vi "Stepper_control_limits.vi"() -> ()   [LabVIEW 2017]
uses:
  <vilib>/Instr/_visa.llb/VISA Configure Serial Port (Instr).vi
panel:
  out "Correction Collar Position":dbl format="%#_3g"
  in  "Load Limits":bool
  in  "Force Stop":bool
  in  "Save Limits":bool
  out "Feedback String":string
  in  "RUN":bool
  in  "Reset Limit":bool
  out "Serial Command":string
  in  "Speed":enum32{"Fine", "Coarse"}(radio)
  in  "Direction":enum32{"Clockwise", "Anticlockwise"}(radio)
  in  "STOP":bool
  out "Second Limit":dbl
  in  "Second Limit":bool
  out "First Limit":dbl
  in  "First Limit":bool
  out "0.17 Position":dbl
  in  "Home":bool
  out "Encoder Position":dbl
  in  "Arduino UNO COM Port":refnum<visa-resource-name>="COM7"
  # "First to Second limit should be set in clockwise sweep"
  # "Do not use unless necessary"
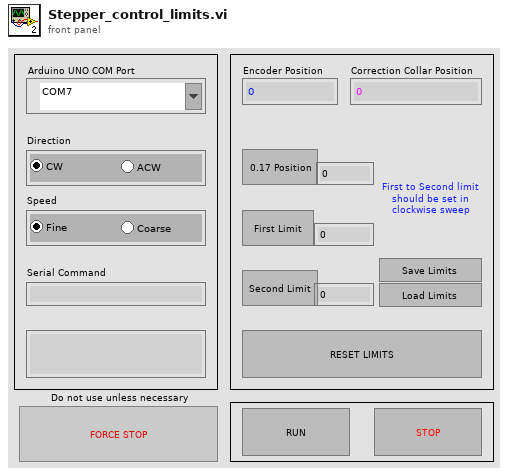
[diagram p1: front panel]
types:
  T1 = enum16{"open", "replace", "create", "open or create", "replace or create", "replace or create with confirmation"}
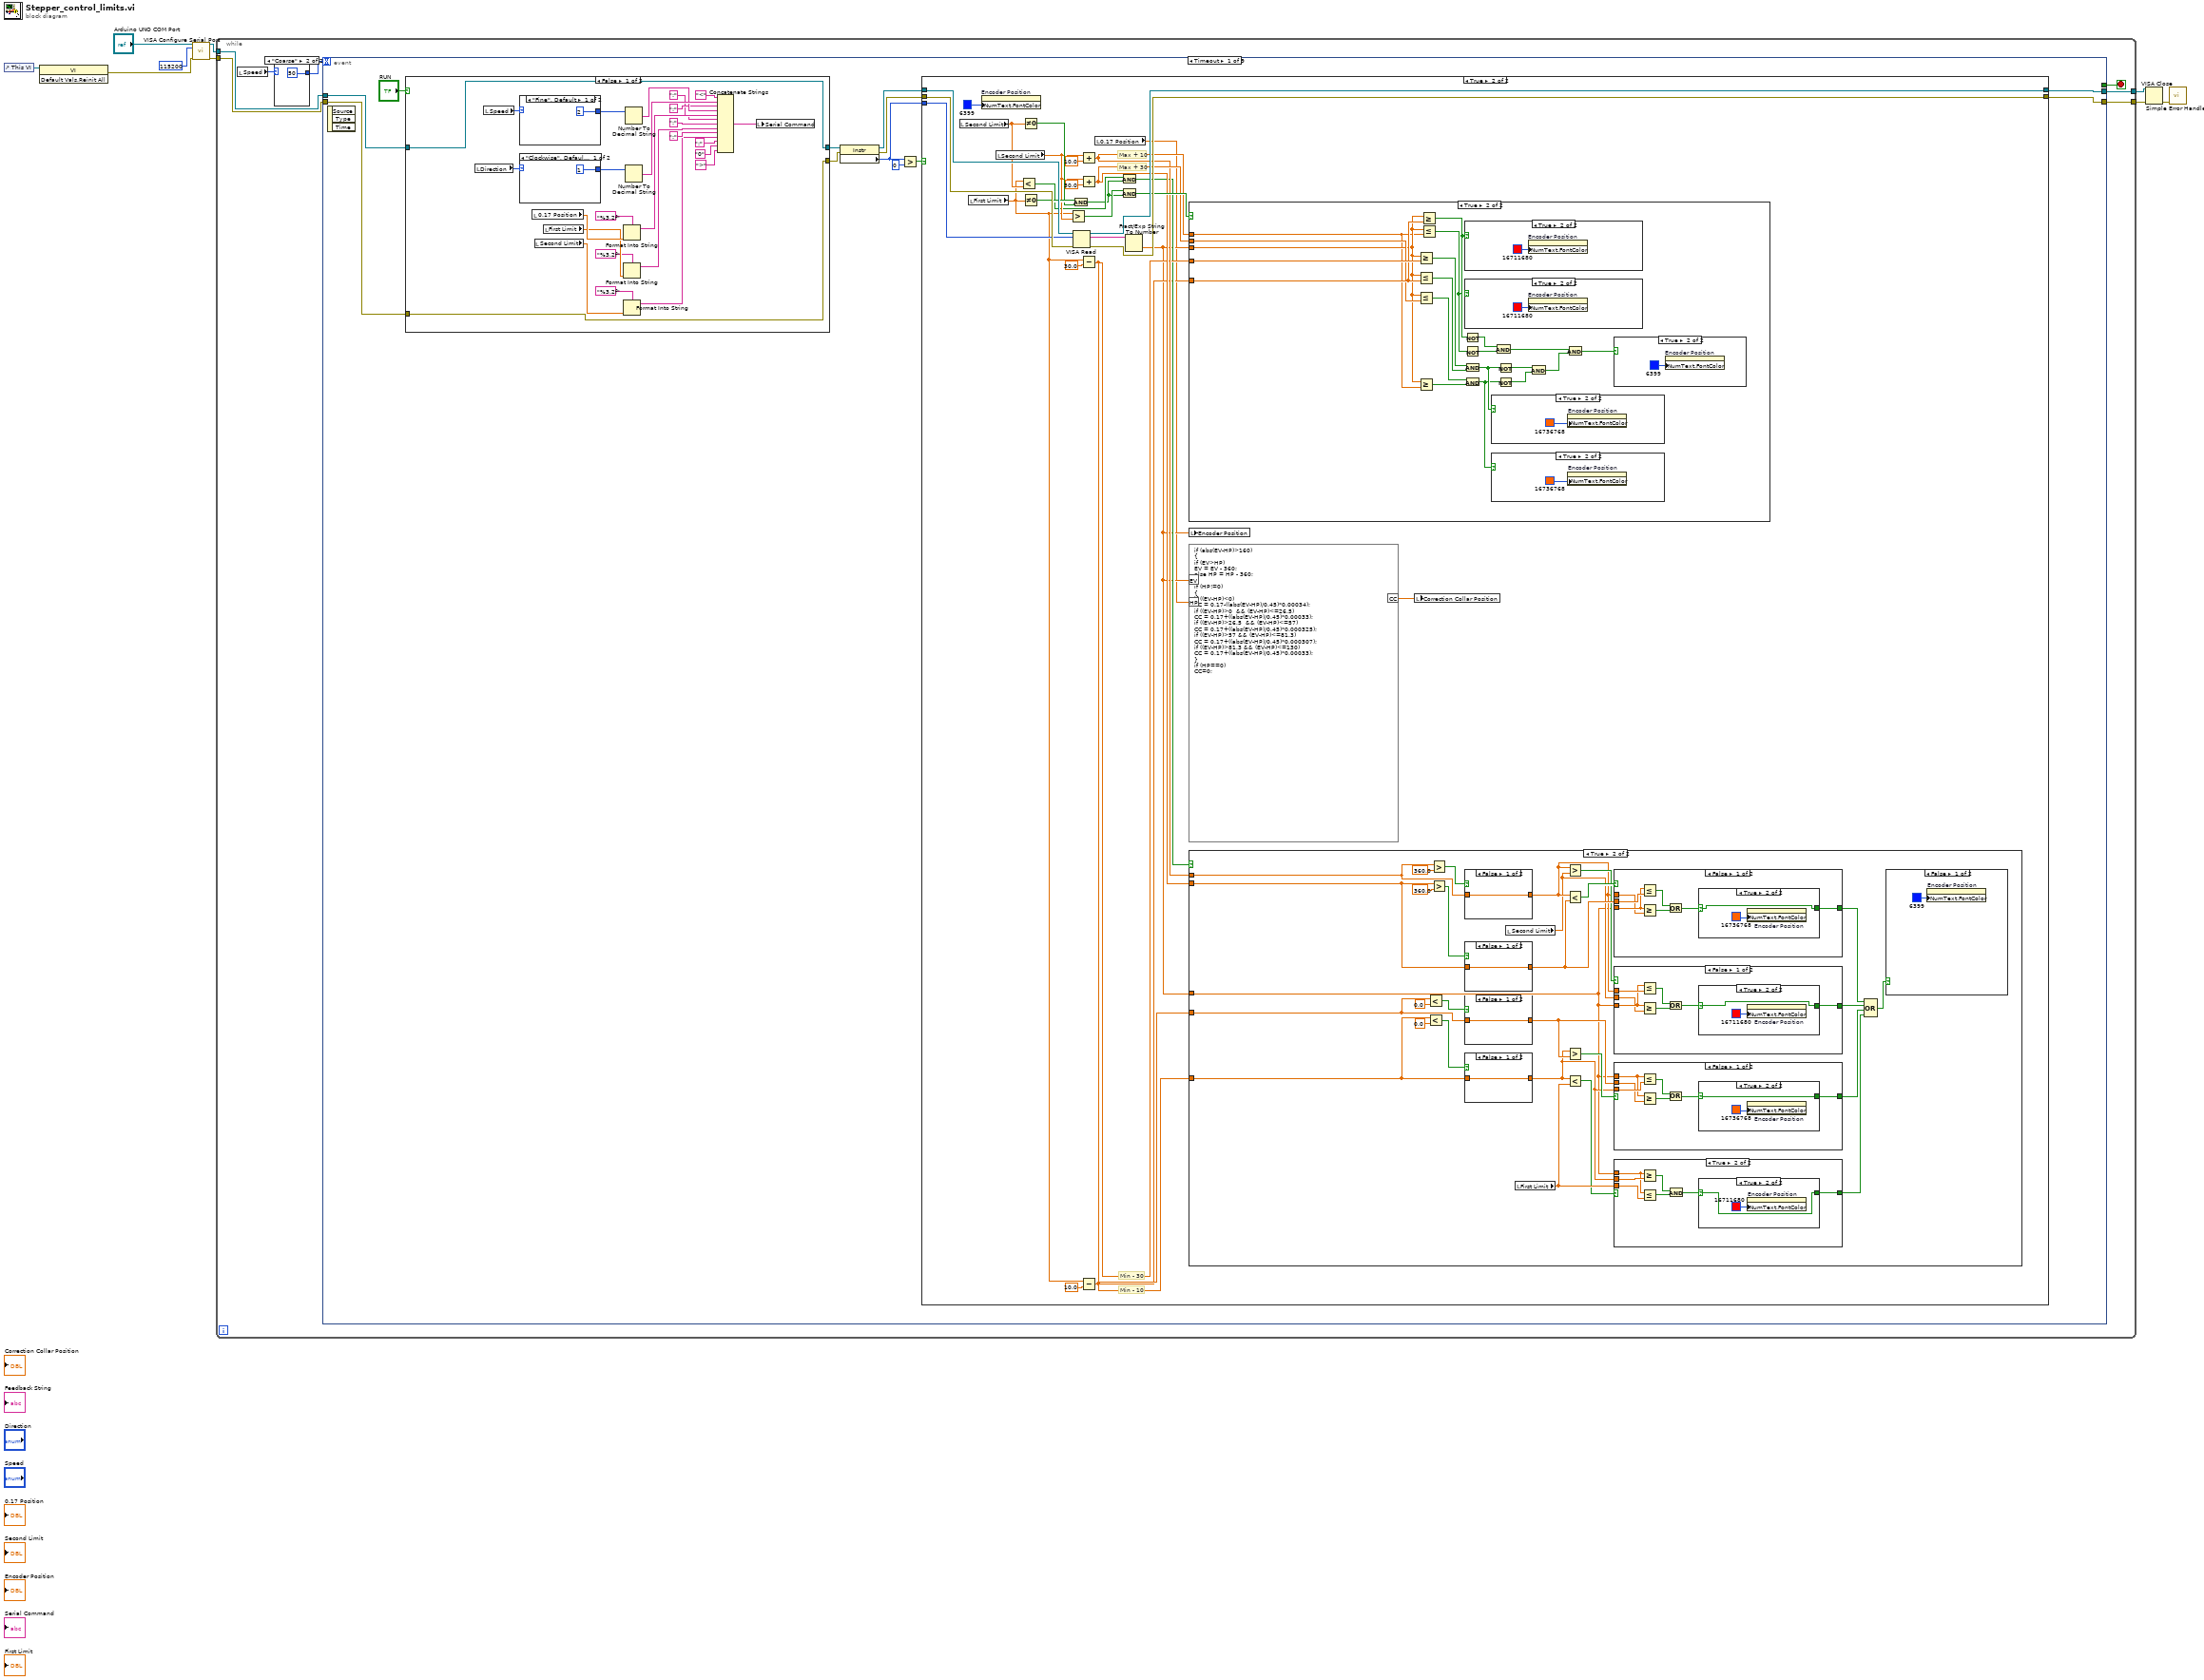
[diagram p0: block diagram]
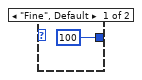
[diagram p2: hidden frame]
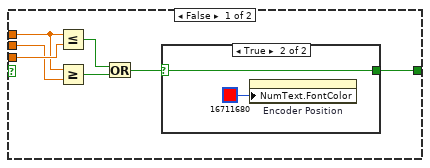
[diagram p6: hidden frame]
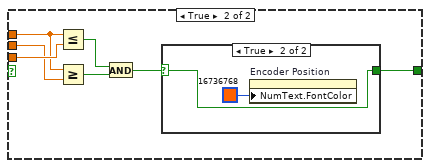
[diagram p10: hidden frame]
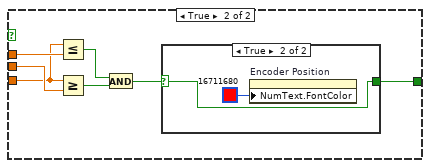
[diagram p13: hidden frame]
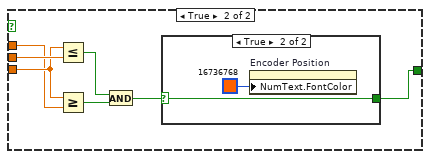
[diagram p16: hidden frame]
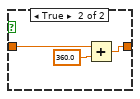
[diagram p18: hidden frame]
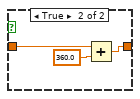
[diagram p19: hidden frame]
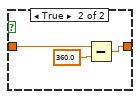
[diagram p20: hidden frame]
diagram:
  n1 = control-ref of="This VI"() -> (w9:refnum<vi>)
  n2 = invoke class="VI" method="Default Vals.Reinit All"(reference=w9) -> (error out=w8:errorcluster)  [unwired: 2 in, 2 out]
  n3 = call-poly "VISA Configure Serial Port"("VISA resource name"="Arduino UNO COM Port", "baud rate (9600)"=u32 115200, "error in (no error)"=w8) -> ("VISA resource name out"=w5:refnum<visa-resource-name>, "error out"=w4:errorcluster)  [unwired: 11 in]
  n4 = while {
    tunnel: w4 -> [w13]
    tunnel: [w11] -> w2
    tunnel: w5 -> [w12]
    tunnel: [w10] -> w3
    stop <- w16 stop-if-true
    n5 = local read "Speed"() -> (w15:enum32{"Fine", "Coarse"})
    n6 = case shown="\"Coarse\"" w15 {
      tunnel: [100 50] -> w14
      frame "Fine", Default {
      }
      frame "Coarse" {
      }
    }
    n7 = event shown="[0] Timeout" {
      selector: _ -> [_ _ _ _ _ _ _ _ _]
      dyn-events: _ -> [_ _ _ _ _ _ _ _ _]
      timeout: w14 -> [_ _ _ _ _ _ _ _ _]
      tunnel: w12 -> [w30 _ w290 w338 _ _ _ _ _]
      tunnel: w13 -> [w29 _ w289 w337 _ _ _ _ _]
      tunnel: [_ _ w293 "Force Stop" _ _ _ _ _] -> w16
      tunnel: [w19 _ w291 w337 _ _ _ _ _] -> w11
      tunnel: [w20 _ w292 w338 _ _ _ _ _] -> w10
      event Timeout {
        n8 = event-data() -> ()  [unwired: 1 in, 3 out]
        n9 = case shown="False" "RUN" {
          tunnel: w30 -> [w222 w268]
          tunnel: w29 -> [w221 w267]
          tunnel: [w222 w266] -> w23
          tunnel: [w221 w265] -> w22
          frame False {
            n10 = local read "Direction"() -> (w232:enum32{"Clockwise", "Anticlockwise"})
            n11 = local read "Speed"() -> (w231:enum32{"Fine", "Coarse"})
            n12 = case shown="\"Fine\", Default" w231 {
              tunnel: [2 1] -> w234
              frame "Fine", Default {
              }
              frame "Coarse" {
              }
            }
            n13 = case shown="\"Clockwise\", Default" w232 {
              tunnel: [1 2] -> w236
              frame "Clockwise", Default {
              }
              frame "Anticlockwise" {
              }
            }
            n14 = local read "0.17 Position"() -> (w218:dbl)
            n15 = local read "Second Limit"() -> (w213:dbl)
            n16 = local read "First Limit"() -> (w216:dbl)
            n17 = Format Into String(format string="%3.2f", w218) -> (resulting string=w219:string)  [unwired: 2 in, 1 out]
            n18 = Format Into String(format string="%3.2f", w216) -> (resulting string=w215:string)  [unwired: 2 in, 1 out]
            n19 = Format Into String(format string="%3.2f", w213) -> (resulting string=w211:string)  [unwired: 2 in, 1 out]
            n20 = Number To Decimal String(number=w234) -> (decimal integer string=w233:string)  [unwired: 1 in]
            n21 = Number To Decimal String(number=w236) -> (decimal integer string=w235:string)  [unwired: 1 in]
            n22 = Concatenate Strings("<" ("string"), w235, ":" ("string"), w233, ":" ("string"), w219, ":" ("string"), w215, ":" ("string"), w211, ":" ("string"), "0" ("string"), ">" ("string")) -> (w220:string)
            n23 = local write "Serial Command"(w220) -> ()
          }
          frame True {
            n24 = local read "Direction"() -> (w252:enum32{"Clockwise", "Anticlockwise"})
            n25 = local read "Speed"() -> (w251:enum32{"Fine", "Coarse"})
            n26 = case shown="\"Fine\", Default" w251 {
              tunnel: [2 1] -> w258
              frame "Fine", Default {
              }
              frame "Coarse" {
              }
            }
            n27 = case shown="\"Clockwise\", Default" w252 {
              tunnel: [1 2] -> w260
              frame "Clockwise", Default {
              }
              frame "Anticlockwise" {
              }
            }
            n28 = local read "0.17 Position"() -> (w249:dbl)
            n29 = local read "Second Limit"() -> (w244:dbl)
            n30 = local read "First Limit"() -> (w246:dbl)
            n31 = Format Into String(format string="%3.2f", w249) -> (resulting string=w247:string)  [unwired: 2 in, 1 out]
            n32 = Format Into String(format string="%3.2f", w246) -> (resulting string=w245:string)  [unwired: 2 in, 1 out]
            n33 = Format Into String(format string="%3.2f", w244) -> (resulting string=w242:string)  [unwired: 2 in, 1 out]
            n34 = Number To Decimal String(number=w258) -> (decimal integer string=w257:string)  [unwired: 1 in]
            n35 = Number To Decimal String(number=w260) -> (decimal integer string=w259:string)  [unwired: 1 in]
            n36 = Concatenate Strings("<" ("string"), w259, ":" ("string"), w257, ":" ("string"), w247, ":" ("string"), w245, ":" ("string"), w242, ":" ("string"), "1" ("string"), ">" ("string")) -> (w250:string)
            n37 = local write "Serial Command"(w250) -> ()
            n38 = VISA Write(VISA resource name=w268, write buffer=w250, error in (no error)=w267) -> (VISA resource name out=w266:refnum<visa-resource-name>, error out=w265:errorcluster)  [unwired: 1 out]
          }
        }
        n39 = property class="Instr"(reference=w23, error in=w22) -> (reference out=w25:refnum<visa-resource-name>, error out=w26:errorcluster, "Serial Settings:Number of Bytes at Serial Port"=w27:u32)
        n40 = Greater?(x=w27, y=u32 0) -> (0:w24:bool)
        n41 = case shown="True" w24 {
          tunnel: [w31 w60] -> w19
          tunnel: [w32 w59] -> w20
          tunnel: w26 -> [w31 w58]
          tunnel: w25 -> [w32 w57]
          tunnel: w27 -> [_ w55]
          frame False {
          }
          frame True {
            # "Min - 30"
            # "Min - 10"
            # "Max + 10"
            # "Max + 30"
            n42 = local read "Second Limit"() -> (w46:dbl)
            n43 = local read "First Limit"() -> (w41:dbl)
            n44 = property on="Encoder Position" class="DigNum (strict)"("NumText.FontColor"=u32 6399) -> ()  [unwired: 2 in, 2 out]
            n45 = local read "Second Limit"() -> (w50:dbl)
            n46 = Less?(x=w41, y=w46) -> (x < y?=w45:bool)
            n47 = Not Equal To 0?(x=w46) -> (x != 0?=w51:bool)
            n48 = Not Equal To 0?(x=w41) -> (x != 0?=w54:bool)
            n49 = Greater?(x=w41, y=w50) -> (0:w53:bool)
            n50 = And(x=w54, y=w51) -> (x .and. y?=w44:bool)
            n51 = VISA Read(VISA resource name=w57, byte count=w55, error in (no error)=w58) -> (VISA resource name out=w59:refnum<visa-resource-name>, read buffer=w56:string, error out=w60:errorcluster)  [unwired: 1 out]
            n52 = Add(x=w50, y=10.0) -> (x+y=w48:dbl)
            n53 = Add(x=w50, y=30.0) -> (x+y=w49:dbl)
            n54 = Subtract(x=w41, y=30.0) -> (x-y=w47:dbl)
            n55 = Subtract(x=w41, y=10.0) -> (x-y=w37:dbl)
            n56 = local read "0.17 Position"() -> (w34:dbl)
            n57 = And(x=w45, y=w44) -> (x .and. y?=w43:bool)
            n58 = And(x=w53, y=w44) -> (x .and. y?=w52:bool)
            n59 = Fract/Exp String To Number(string=w56) -> (number=w35:dbl)  [unwired: 3 in, 1 out]
            n60 = case shown="True" w52 {
              tunnel: w35 -> [_ w198]
              tunnel: w47 -> [_ w205]
              tunnel: w37 -> [_ w202]
              tunnel: w49 -> [_ w201]
              tunnel: w48 -> [_ w197]
              frame False {
              }
              frame True {
                n61 = Greater Or Equal?(x=w198, y=w205) -> (x >= y?=w204:bool)
                n62 = Less Or Equal?(x=w198, y=w202) -> (x <= y?=w203:bool)
                n63 = Less Or Equal?(x=w198, y=w201) -> (x <= y?=w200:bool)
                n64 = Greater Or Equal?(x=w198, y=w197) -> (x >= y?=w199:bool)
                n65 = Greater Or Equal?(x=w198, y=w202) -> (x >= y?=w193:bool)
                n66 = Less Or Equal?(x=w198, y=w197) -> (x <= y?=w192:bool)
                n67 = Not(x=w193) -> (.not. x?=w190:bool)
                n68 = Not(x=w192) -> (.not. x?=w191:bool)
                n69 = And(x=w204, y=w203) -> (x .and. y?=w189:bool)
                n70 = And(x=w200, y=w199) -> (x .and. y?=w188:bool)
                n71 = case shown="True" w193 {
                  frame False {
                  }
                  frame True {
                    n72 = property on="Encoder Position" class="DigNum (strict)"("NumText.FontColor"=u32 16711680) -> ()  [unwired: 2 in, 2 out]
                  }
                }
                n73 = case shown="True" w192 {
                  frame False {
                  }
                  frame True {
                    n74 = property on="Encoder Position" class="DigNum (strict)"("NumText.FontColor"=u32 16711680) -> ()  [unwired: 2 in, 2 out]
                  }
                }
                n75 = case shown="True" w189 {
                  frame False {
                  }
                  frame True {
                    n76 = property on="Encoder Position" class="DigNum (strict)"("NumText.FontColor"=u32 16736768) -> ()  [unwired: 2 in, 2 out]
                  }
                }
                n77 = case shown="True" w188 {
                  frame False {
                  }
                  frame True {
                    n78 = property on="Encoder Position" class="DigNum (strict)"("NumText.FontColor"=u32 16736768) -> ()  [unwired: 2 in, 2 out]
                  }
                }
                n79 = And(x=w190, y=w191) -> (x .and. y?=w196:bool)
                n80 = Not(x=w189) -> (.not. x?=w187:bool)
                n81 = Not(x=w188) -> (.not. x?=w186:bool)
                n82 = And(x=w187, y=w186) -> (x .and. y?=w195:bool)
                n83 = And(x=w196, y=w195) -> (x .and. y?=w194:bool)
                n84 = case shown="True" w194 {
                  frame False {
                  }
                  frame True {
                    n85 = property on="Encoder Position" class="DigNum (strict)"("NumText.FontColor"=u32 6399) -> ()  [unwired: 2 in, 2 out]
                  }
                }
              }
            }
            n86 = local write "Encoder Position"(w35) -> ()
            n87 = formula code="if (abs(EV-HP)>160)\n{\nif (EV>HP)\nEV = EV - 360;\nelse HP = HP - 360;\n}\nif (HP!=0)\n{\nif ((EV-HP)<0)\nCC = 0.17-((abs(EV-HP)/0.45)*0.00034);\nif ((EV-HP)>0  && (EV-HP)<=26.5)\nCC = 0.17+((abs(EV-HP)/0.45)*0.00033);\nif ((EV-HP)>26.5  && (EV-HP)<=57)\nCC = 0.17+((abs(EV-HP)/0.45)*0.000325);\nif ((EV-HP)>57 && (EV-HP)<=81.3)\nCC = 0.17+((abs(EV-HP)/0.45)*0.000307);\nif ((EV-HP)>81.3 && (EV-HP)<=130)\nCC = 0.17+((abs(EV-HP)/0.45)*0.00033);\n}\nif (HP==0)\nCC=0;"("EV"=w35, "HP"=w34) -> ("CC"=w33:dbl)
            n88 = case shown="True" w43 {
              tunnel: w35 -> [_ w68]
              tunnel: w49 -> [_ w84]
              tunnel: w48 -> [_ w83]
              tunnel: w47 -> [_ w77]
              tunnel: w37 -> [_ w78]
              frame False {
              }
              frame True {
                n89 = Less?(x=w77, y=0.0) -> (x < y?=w80:bool)
                n90 = Less?(x=w78, y=0.0) -> (x < y?=w79:bool)
                n91 = Greater?(x=w83, y=360.0) -> (0:w86:bool)
                n92 = Greater?(x=w84, y=360.0) -> (0:w85:bool)
                n93 = case shown="False" w86 {
                  tunnel: w83 -> [w182 w185]
                  tunnel: [w182 w183] -> w73
                  frame False {
                  }
                  frame True {
                    n94 = Subtract(x=w185, y=360.0) -> (x-y=w183:dbl)
                  }
                }
                n95 = case shown="False" w85 {
                  tunnel: w84 -> [w178 w180]
                  tunnel: [w178 w179] -> w75
                  frame False {
                  }
                  frame True {
                    n96 = Subtract(x=w180, y=360.0) -> (x-y=w179:dbl)
                  }
                }
                n97 = case shown="False" w80 {
                  tunnel: w77 -> [w174 w177]
                  tunnel: [w174 w175] -> w70
                  frame False {
                  }
                  frame True {
                    n98 = Add(x=w177, y=360.0) -> (x+y=w175:dbl)
                  }
                }
                n99 = case shown="False" w79 {
                  tunnel: w78 -> [w170 w172]
                  tunnel: [w170 w171] -> w69
                  frame False {
                  }
                  frame True {
                    n100 = Add(x=w172, y=360.0) -> (x+y=w171:dbl)
                  }
                }
                n101 = local read "Second Limit"() -> (w72:dbl)
                n102 = local read "First Limit"() -> (w67:dbl)
                n103 = Greater?(x=w73, y=w72) -> (0:w74:bool)
                n104 = Less?(x=w73, y=w75) -> (x < y?=w76:bool)
                n105 = Greater?(x=w69, y=w70) -> (0:w71:bool)
                n106 = Less?(x=w69, y=w67) -> (x < y?=w66:bool)
                n107 = case shown="False" w76 {
                  tunnel: w68 -> [w155 w165]
                  tunnel: w73 -> [w154 w164]
                  tunnel: w75 -> [w156 w166]
                  tunnel: [w150 w160] -> w65
                  frame False {
                    n108 = Less Or Equal?(x=w155, y=w156) -> (x <= y?=w153:bool)
                    n109 = Greater Or Equal?(x=w155, y=w154) -> (x >= y?=w152:bool)
                    n110 = Or(x=w153, y=w152) -> (x .or. y?=w151:bool)
                    n111 = case shown="True" w151 {
                      selector: w151 -> [w157 w158]
                      tunnel: [w157 w158] -> w150
                      frame False {
                      }
                      frame True {
                        n112 = property on="Encoder Position" class="DigNum (strict)"("NumText.FontColor"=u32 16736768) -> ()  [unwired: 2 in, 2 out]
                      }
                    }
                  }
                  frame True {
                    n113 = Less Or Equal?(x=w165, y=w166) -> (x <= y?=w163:bool)
                    n114 = Greater Or Equal?(x=w165, y=w164) -> (x >= y?=w162:bool)
                    n115 = And(x=w163, y=w162) -> (x .and. y?=w161:bool)
                    n116 = case shown="True" w161 {
                      selector: w161 -> [w167 w168]
                      tunnel: [w167 w168] -> w160
                      frame False {
                      }
                      frame True {
                        n117 = property on="Encoder Position" class="DigNum (strict)"("NumText.FontColor"=u32 16736768) -> ()  [unwired: 2 in, 2 out]
                      }
                    }
                  }
                }
                n118 = case shown="False" w74 {
                  tunnel: w68 -> [w135 w143]
                  tunnel: w73 -> [w136 w146]
                  tunnel: w72 -> [w134 w144]
                  tunnel: [w130 w145] -> w64
                  frame False {
                    n119 = Less Or Equal?(x=w135, y=w136) -> (x <= y?=w133:bool)
                    n120 = Greater Or Equal?(x=w135, y=w134) -> (x >= y?=w132:bool)
                    n121 = Or(x=w133, y=w132) -> (x .or. y?=w131:bool)
                    n122 = case shown="True" w131 {
                      selector: w131 -> [w137 w138]
                      tunnel: [w137 w138] -> w130
                      frame False {
                      }
                      frame True {
                        n123 = property on="Encoder Position" class="DigNum (strict)"("NumText.FontColor"=u32 16711680) -> ()  [unwired: 2 in, 2 out]
                      }
                    }
                  }
                  frame True {
                    n124 = Less Or Equal?(x=w143, y=w146) -> (x <= y?=w142:bool)
                    n125 = Greater Or Equal?(x=w143, y=w144) -> (x >= y?=w141:bool)
                    n126 = And(x=w142, y=w141) -> (x .and. y?=w140:bool)
                    n127 = case shown="True" w140 {
                      selector: w140 -> [w147 w148]
                      tunnel: [w147 w148] -> w145
                      frame False {
                      }
                      frame True {
                        n128 = property on="Encoder Position" class="DigNum (strict)"("NumText.FontColor"=u32 16711680) -> ()  [unwired: 2 in, 2 out]
                      }
                    }
                  }
                }
                n129 = case shown="False" w71 {
                  tunnel: w68 -> [w115 w125]
                  tunnel: w69 -> [w116 w126]
                  tunnel: w70 -> [w114 w124]
                  tunnel: [w110 w120] -> w63
                  frame False {
                    n130 = Less Or Equal?(x=w115, y=w116) -> (x <= y?=w112:bool)
                    n131 = Greater Or Equal?(x=w115, y=w114) -> (x >= y?=w113:bool)
                    n132 = Or(x=w112, y=w113) -> (x .or. y?=w111:bool)
                    n133 = case shown="True" w111 {
                      selector: w111 -> [w117 w118]
                      tunnel: [w117 w118] -> w110
                      frame False {
                      }
                      frame True {
                        n134 = property on="Encoder Position" class="DigNum (strict)"("NumText.FontColor"=u32 16736768) -> ()  [unwired: 2 in, 2 out]
                      }
                    }
                  }
                  frame True {
                    n135 = Less Or Equal?(x=w125, y=w126) -> (x <= y?=w123:bool)
                    n136 = Greater Or Equal?(x=w125, y=w124) -> (x >= y?=w122:bool)
                    n137 = And(x=w123, y=w122) -> (x .and. y?=w121:bool)
                    n138 = case shown="True" w121 {
                      selector: w121 -> [w127 w128]
                      tunnel: [w127 w128] -> w120
                      frame False {
                      }
                      frame True {
                        n139 = property on="Encoder Position" class="DigNum (strict)"("NumText.FontColor"=u32 16736768) -> ()  [unwired: 2 in, 2 out]
                      }
                    }
                  }
                }
                n140 = case shown="True" w66 {
                  tunnel: w69 -> [w94 w106]
                  tunnel: w68 -> [w95 w104]
                  tunnel: w67 -> [w96 w103]
                  tunnel: [w90 w105] -> w62
                  frame False {
                    n141 = Less Or Equal?(x=w95, y=w96) -> (x <= y?=w93:bool)
                    n142 = Greater Or Equal?(x=w95, y=w94) -> (x >= y?=w92:bool)
                    n143 = Or(x=w93, y=w92) -> (x .or. y?=w91:bool)
                    n144 = case shown="True" w91 {
                      selector: w91 -> [w97 w98]
                      tunnel: [w97 w98] -> w90
                      frame False {
                      }
                      frame True {
                        n145 = property on="Encoder Position" class="DigNum (strict)"("NumText.FontColor"=u32 16711680) -> ()  [unwired: 2 in, 2 out]
                      }
                    }
                  }
                  frame True {
                    n146 = Greater Or Equal?(x=w104, y=w106) -> (x >= y?=w101:bool)
                    n147 = Less Or Equal?(x=w104, y=w103) -> (x <= y?=w100:bool)
                    n148 = And(x=w101, y=w100) -> (x .and. y?=w102:bool)
                    n149 = case shown="True" w102 {
                      selector: w102 -> [w107 w108]
                      tunnel: [w107 w108] -> w105
                      frame False {
                      }
                      frame True {
                        n150 = property on="Encoder Position" class="DigNum (strict)"("NumText.FontColor"=u32 16711680) -> ()  [unwired: 2 in, 2 out]
                      }
                    }
                  }
                }
                n151 = Compound Arithmetic op=OR(w65, w64, w63, w62) -> (w61:bool)
                n152 = case shown="False" w61 {
                  frame False {
                    n153 = property on="Encoder Position" class="DigNum (strict)"("NumText.FontColor"=u32 6399) -> ()  [unwired: 2 in, 2 out]
                  }
                  frame True {
                  }
                }
              }
            }
            n154 = local write "Correction Collar Position"(w33) -> ()
          }
        }
      }
      event "Load Limits": Value Change {
        n155 = event-data() -> ()  [unwired: 1 in, 6 out]
        n156 = call <vilib>:"Dflt Data Dir.vi"() -> ("App:Default Data Directory"=w282:path)
        n157 = Build Path(base path=w282, name or relative path=path "limits.txt" ("default name")) -> (appended path=w283:path)
        n158 = local write "Feedback String"("Limits loaded!" ("Feedback String")) -> ()
        n159 = Read from Text File(file (use dialog)=w283) -> (text=w284:string)  [unwired: 2 in, 4 out]
        n160 = Spreadsheet String To Array(format string="%.2f", spreadsheet string=w284) -> (array=w285:dbl[][])  [unwired: 2 in]
        n161 = Index Array(array=w285, index (row) #1=0 ("disabled index (row)"), index (col) #1=0 ("disabled index (col)"), index (row) #2=0 ("disabled index (row)"), index (col) #2=1 ("disabled index (col)"), index (row) #3=0 ("disabled index (row)"), index (col) #3=2 ("disabled index (col)")) -> (element #1=w286:dbl, element #2=w287:dbl, element #3=w288:dbl)
        n162 = local write "First Limit"(w286) -> ()
        n163 = local write "0.17 Position"(w287) -> ()
        n164 = local write "Second Limit"(w288) -> ()
      }
      event "STOP": Value Change {
        n165 = event-data() -> ()  [unwired: 1 in, 6 out]
        n166 = case shown="True" "STOP" {
          tunnel: [FALSE w312] -> w293
          tunnel: w290 -> [w296 w311]
          tunnel: w289 -> [w295 w310]
          tunnel: [w296 w309] -> w292
          tunnel: [w295 w308] -> w291
          frame False {
          }
          frame True {
            w305 = 0.0 ("y")
            n167 = local read "Second Limit"() -> (w306:dbl)
            n168 = local read "First Limit"() -> (w307:dbl)
            n169 = local read "0.17 Position"() -> (w304:dbl)
            n170 = Equal?(x=w307, y=w305) -> (x = y?=w303:bool)
            n171 = Equal?(x=w306, y=w305) -> (x = y?=w302:bool)
            n172 = Or(x=w303, y=w302) -> (x .or. y?=w300:bool)
            n173 = Equal?(x=w304, y=w305) -> (x = y?=w301:bool)
            n174 = And(x=w300, y=w301) -> (x .and. y?=w299:bool)
            n175 = Not(x=w299) -> (.not. x?=w298:bool)
            n176 = case shown="True" w298 {
              tunnel: [TRUE w320] -> w312
              tunnel: w311 -> [w315 w319]
              tunnel: w310 -> [w314 w318]
              tunnel: [w315 w317] -> w309
              tunnel: [w314 w316] -> w308
              frame False {
              }
              frame True {
                n177 = local read "Encoder Position"() -> (w326:dbl)
                n178 = local read "0.17 Position"() -> (w325:dbl)
                n179 = Subtract(x=w326, y=w325) -> (x-y=w324:dbl)
                n180 = Absolute Value(x=w324) -> (abs(x)=w323:dbl)
                n181 = Less?(x=w323, y=10.0) -> (x < y?=w321:bool)
                n182 = case shown="False" w321 {
                  tunnel: [FALSE TRUE] -> w320
                  tunnel: w319 -> [w330 w334]
                  tunnel: w318 -> [w329 w333]
                  tunnel: [w330 w332] -> w317
                  tunnel: [w329 w331] -> w316
                  frame False {
                    n183 = One Button Dialog(message="Encoder Value should be less than 10 degrees of 0.17 (Home) Position") -> ()  [unwired: 1 in, 1 out]
                  }
                  frame True {
                    w335 = ":" ("write buffer")
                    n184 = local write "Serial Command"(w335) -> ()
                    n185 = VISA Write(VISA resource name=w334, write buffer=w335, error in (no error)=w333) -> (VISA resource name out=w332:refnum<visa-resource-name>, error out=w331:errorcluster)  [unwired: 1 out]
                  }
                }
              }
            }
          }
        }
      }
      event "Force Stop": Value Change {
        n186 = event-data() -> ()  [unwired: 1 in, 6 out]
      }
      event "First Limit": Value Change {
        n187 = event-data() -> ()  [unwired: 1 in, 6 out]
        n188 = local read "Encoder Position"() -> (w341:dbl)
        n189 = local write "First Limit"(w341) -> ()
        n190 = local write "Feedback String"("First Limit set! \nCW--> Fine ---> RUN to set second limit!!" ("Feedback String")) -> ()
      }
      event "Second Limit": Value Change {
        n191 = event-data() -> ()  [unwired: 1 in, 6 out]
        n192 = local read "Encoder Position"() -> (w343:dbl)
        n193 = local write "Second Limit"(w343) -> ()
        n194 = local write "Feedback String"("Second Limit set!\n" ("Feedback String")) -> ()
      }
      event "Home": Value Change {
        n195 = event-data() -> ()  [unwired: 1 in, 6 out]
        n196 = local write "Correction Collar Position"(0.17 ("Correction Collar Position")) -> ()
        n197 = local read "Encoder Position"() -> (w346:dbl)
        n198 = local write "0.17 Position"(w346) -> ()
        n199 = local write "Feedback String"("0.17 Position set!" ("Feedback String")) -> ()
      }
      event "Save Limits": Value Change {
        n200 = event-data() -> ()  [unwired: 1 in, 6 out]
        n201 = local read "0.17 Position"() -> (w362:dbl)
        n202 = local read "Second Limit"() -> (w361:dbl)
        n203 = local read "First Limit"() -> (w363:dbl)
        n204 = call <vilib>:"Dflt Data Dir.vi"() -> ("App:Default Data Directory"=w347:path)
        n205 = Build Array(w363, w362, w361) -> (w355:dbl[])
        n206 = Build Path(base path=w347, name or relative path=path "limits.txt" ("default name")) -> (appended path=w358:path)
        n207 = Array To Spreadsheet String(array=w355, 3:"%.2f" ("format string")) -> (spreadsheet string=w353:string)  [unwired: 1 out]
        n208 = Open/Create/Replace File(file path (use dialog)=w358, operation (0:open)=T1."replace or create with confirmation", access (0:read/write)=enum16{"read/write", "read-only", "write-only"}."read/write") -> (refnum out=w352:refnum<file>, error out=w351:errorcluster)  [unwired: 1 in, 3 out]
        n209 = local write "Feedback String"("Limits saved in 'limits.txt' in Labview data path." ("Feedback String")) -> ()
        n210 = Write to Text File(file (use dialog)=w352, text=w353, error in=w351) -> (refnum out=w350:refnum<file>, error out=w349:errorcluster)  [unwired: 1 in, 1 out]
        n211 = Close File(refnum=w350, error in=w349) -> (error out=w348:errorcluster)  [unwired: 1 out]
        n212 = call <vilib>:"Simple Error Handler.vi"("error in (no error)"=w348) -> ()  [unwired: 1 in, 8 out]
      }
      event "Reset Limit": Value Change {
        n213 = event-data() -> ()  [unwired: 1 in, 6 out]
        n214 = local write "Second Limit"(0.0 ("Maximum Limit")) -> ()
        n215 = local write "First Limit"(0.0 ("Minimum Limit")) -> ()
        n216 = local write "0.17 Position"(0.0 ("Home Position")) -> ()
        n217 = local read "Direction"() -> (w376:enum32{"Clockwise", "Anticlockwise"})
        n218 = local read "Speed"() -> (w373:enum32{"Fine", "Coarse"})
        n219 = case shown="\"Fine\", Default" w373 {
          tunnel: [2 1] -> w372
          frame "Fine", Default {
          }
          frame "Coarse" {
          }
        }
        n220 = case shown="\"Clockwise\", Default" w376 {
          tunnel: [1 2] -> w375
          frame "Clockwise", Default {
          }
          frame "Anticlockwise" {
          }
        }
        n221 = Number To Decimal String(number=w372) -> (decimal integer string=w371:string)  [unwired: 1 in]
        n222 = Number To Decimal String(number=w375) -> (decimal integer string=w374:string)  [unwired: 1 in]
        n223 = Concatenate Strings("<" ("string"), w374, ":" ("string"), w371, ":" ("string"), "0" ("string"), ":" ("string"), "0" ("string"), ":" ("string"), "0" ("string"), ":" ("string"), "0" ("string"), ">" ("string")) -> (w384:string)
        n224 = local write "Serial Command"(w384) -> ()
      }
    }
  }
  n225 = VISA Close(VISA resource name=w3, error in (no error)=w2) -> (error out=w1:errorcluster)
  n226 = call <vilib>:"Simple Error Handler.vi"("error in (no error)"=w1) -> ()  [unwired: 4 in, 5 out]
